vi "DrawLine.vi"(6 "color(black)":u32, 7 "offset":cluster{"X":dbl, "Y":dbl}, 9 "move":cluster{dbl, dbl}, 10 "start":cluster{"a":dbl, dbl}, 11 "picture in":picture) -> (3 "picture out":picture)   [LabVIEW 2020]
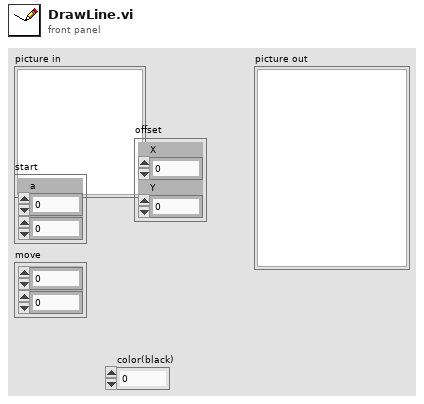
[diagram p1: front panel]
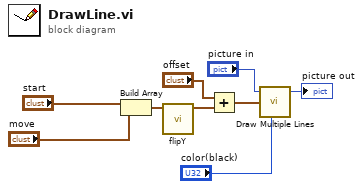
[diagram p0: block diagram]
diagram:
  n1 = Build Array("start", "move") -> (w7:cluster{"a":dbl, dbl}[])
  n2 = call "flipY.vi"("Array in"=w7) -> ("Array out"=w6:cluster{"a":dbl, dbl}[])  [unwired: 10 in]
  n3 = Add(x="offset", y=w6) -> (x+y=w5:cluster{dbl, dbl}[])
  n4 = call <vilib>:"Draw Multiple Lines.vi"("picture"="picture in", "line endpoints"=w5, "color(black)"="color(black)") -> ("new picture"=→"picture out":picture)  [unwired: 6 in]
